vi "IMAQdx LL-Sequence.vi"(8 "ErrIn":errorcluster) -> (0 "ErrOut":errorcluster)   [LabVIEW 2013]
doc: "Use this template to build a VI to use as a subVI."
uses:
  <vilib>/vision/Image Controls.llb/IMAQ Image.ctl
  <vilib>/vision/driver/IMAQdx.llb/IMAQdx Acquisition Mode.ctl
  <vilib>/vision/driver/IMAQdx.llb/IMAQdx Buffer Number Mode.ctl
  <vilib>/vision/driver/NI_Vision_Acquisition_Software.lvlib
panel:
  in  "Camera":refnum<k21> caption="IMAQdx Session"
  out "ImgOut":T1[](array[typedef])
  in  "Number of images":i32=10
  # "Input Parameters"
  # "Output Parameters"
  # "VI Description:\nLow Level IMAQ Sequence"
  # ":: MVI Framework V1.0 ::\nAuthor:Gaoke Yang\nEmail: gaoke.yang@yahoo.com\nWeb: www.mvicontrol.com\nCopyright (C) 2013, MVI Technologies All Rights Reserved"
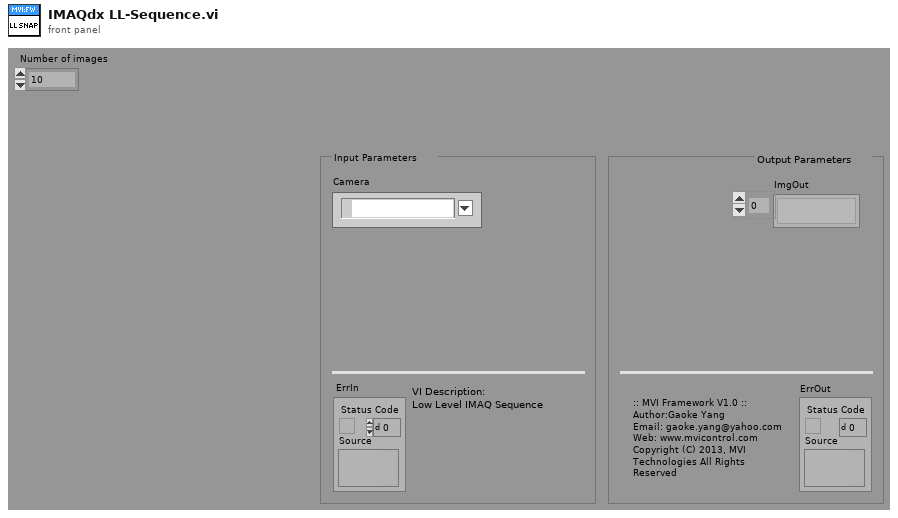
[diagram p1: front panel]
types:
  T1 = typedef "IMAQ Image.ctl" = refnum<image>
  T2 = typedef "NI_Vision_Acquisition_Software.lvlib/IMAQdx Buffer Number Mode.ctl" = enum32{"Next", "Last", "Buffer Number"}
  T3 = typedef "NI_Vision_Acquisition_Software.lvlib/IMAQdx Acquisition Mode.ctl" = enum32{"One Shot", "Continuous"}
  T4 = typedef "IMAQdx.ctl" = refnum<k21>
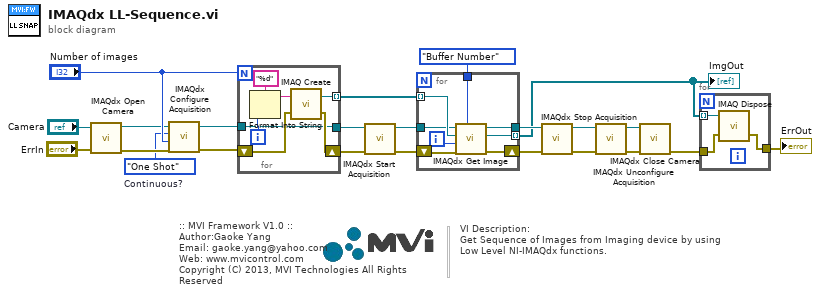
[diagram p0: block diagram]
diagram:
  w17 = IMAQdx_Acquisition_Mode."One Shot"  # Continuous?
  # "VI Description:\nGet Sequence of Images from Imaging device by using \nLow Level NI-IMAQdx functions."
  # ":: MVI Framework V1.0 ::\nAuthor:Gaoke Yang\nEmail: gaoke.yang@yahoo.com\nWeb: www.mvicontrol.com\nCopyright (C) 2013, MVI Technologies All Rights Reserved"
  n1 = call <vilib>:"IMAQdx Open Camera.vi"("error in"="ErrIn", "Session In"="Camera") -> ("error out"=w19:errorcluster, "Session Out"=w18:T4)  [unwired: 8 in]
  n2 = call <vilib>:"IMAQdx Configure Acquisition.vi"("error in"=w19, "Number of Buffers"="Number of images", "Continuous?"=w17, "Session In"=w18) -> ("error out"=w2:errorcluster, "Session Out"=w16:T4)  [unwired: 6 in]
  n3 = for {
    N: "Number of images" -> [_]
    shift-right: [w26] -> w14
    shift-left: w2 -> [w30]
    tunnel: [w25] -> w20 mode=indexing
    tunnel: w16 -> [w24]
    tunnel: [w24] -> w15
    i -> [w27]
    n4 = Format Into String(format string="%d", w27) -> (resulting string=w29:string)  [unwired: 2 in, 1 out]
    n5 = call "IMAQ Create"("Image Name"=w29, "error in (no error)"=w30) -> ("New Image"=w25:T1, "error out"=w26:errorcluster)  [unwired: 2 in, 1 out]
  }
  n6 = call <vilib>:"IMAQdx Start Acquisition.vi"("error in"=w14, "Session In"=w15) -> ("error out"=w13:errorcluster, "Session Out"=w12:T4)  [unwired: 8 in]
  n7 = for {
    tunnel: [w38] -> w6
    shift-right: [w37] -> w5
    shift-left: w13 -> [w35]
    tunnel: w20 -> [w34] mode=indexing
    tunnel: w12 -> [w33]
    tunnel: IMAQdx_Buffer_Number_Mode."Buffer Number" ("Buffer Number Mode (Next)") -> [w32]
    tunnel: [w31] -> w3 mode=indexing
    i -> [w36]
    n8 = call <vilib>:"IMAQdx Get Image.vi"("Buffer Number Mode (Next)"=w32, "error in"=w35, "Buffer Number In"=w36, "Image In"=w34, "Session In"=w33) -> ("error out"=w37:errorcluster, "Image Out"=w31:T1, "Session Out"=w38:T4)  [unwired: 3 in, 1 out]
  }
  "ImgOut" <- w3
  n9 = call <vilib>:"IMAQdx Stop Acquisition.vi"("error in"=w5, "Session In"=w6) -> ("error out"=w9:errorcluster, "Session Out"=w10:T4)  [unwired: 8 out]
  n10 = call <vilib>:"IMAQdx Unconfigure Acquisition.vi"("error in"=w9, "Session In"=w10) -> ("error out"=w8:errorcluster, "Session Out"=w7:T4)  [unwired: 8 out]
  n11 = call <vilib>:"IMAQdx Close Camera.vi"("error in"=w8, "Session In"=w7) -> ("error out"=w4:errorcluster)  [unwired: 9 out]
  n12 = for {
    tunnel: w4 -> [w40]
    tunnel: w3 -> [w41] mode=indexing
    tunnel: [w39] -> w21
    n13 = call "IMAQ Dispose"("Image"=w41, "error in (no error)"=w40) -> ("error out"=w39:errorcluster)  [unwired: 1 in, 3 out]
  }
  "ErrOut" <- w21
